vi "From Variant.vi"(0 "TTLController in":refnum<class "TTLController.lvclass">, 7 "Variant":variant, 9 "Prefix":string, 11 "error in (no error)":errorcluster) -> (4 "TTLController out":refnum<class "TTLController.lvclass">, 15 "error out":errorcluster)   [LabVIEW 2020, in "TTLController.lvclass"]
uses:
  TTLController.lvclass
  D:/Experiment VIs/Koop/KObject Class/KObject.lvclass
  epl-vi-lib/Koop/KObject Class/KObject.lvclass/KObject.ctl
  TTLController.lvclass/TTLController.ctl
  V0.ctl
  V2.ctl
  Trigger.ctl
  epl-vi-lib/Koop/KObject Class/Read Version.vi
  epl-vi-lib/Koop/KObject Class/KObject.lvclass
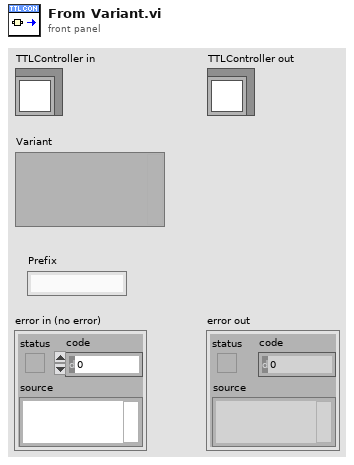
[diagram p1: front panel]
types:
  T1 = typedef "TTLController.lvclass/Serialized.ctl" = cluster{"Name":string, "Start":T2, "Stop":T2, "Pulse":cluster{"Active":bool, "IPI":string, "Width (ms)":dbl}}
  T2 = typedef "TTLController.lvclass/Trigger.ctl" = cluster{"When":string, "Expr":string}
  T3 = typedef "TTLController.lvclass/V0.ctl" = cluster{"Name":string, "Start":cluster{"When":string, "Value":dbl}, "Stop":cluster{"When":string, "Value":dbl}, "Pulse":cluster{"Active":bool, "Rate (Hz)":dbl, "Width (ms)":dbl}}
  T4 = typedef "TTLController.lvclass/V2.ctl" = cluster{"Name":string, "Start":T2, "Stop":T2, "Pulse":cluster{"Active":bool, "Rate (Hz)":dbl, "Width (ms)":dbl}}
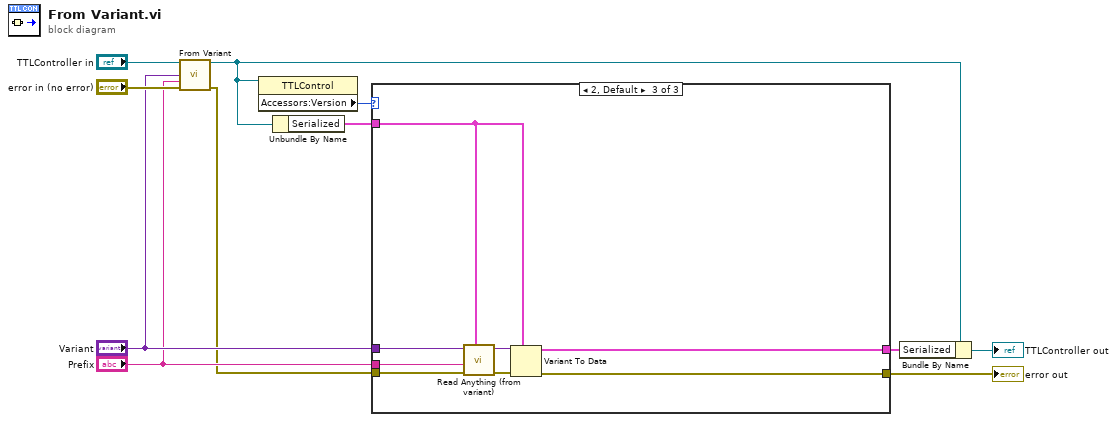
[diagram p0: block diagram]
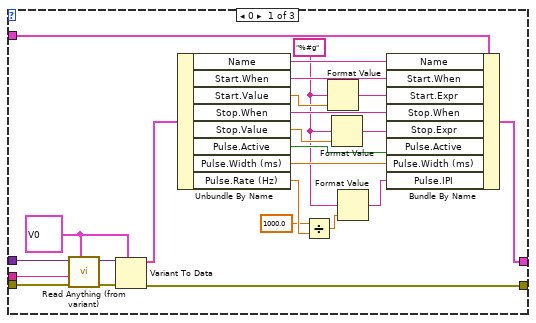
[diagram p2: hidden frame]
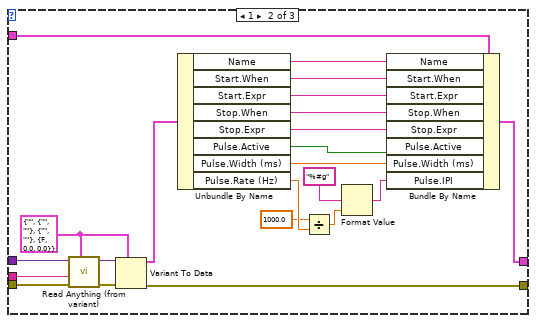
[diagram p3: hidden frame]
diagram:
  n1 = call-parent "From Variant.vi"("KObject in"="TTLController in", "Variant"="Variant", "Prefix"="Prefix", "error in (no error)"="error in (no error)") -> ("KObject out"=w2:refnum<class "TTLController.lvclass">, "error out"=w6:errorcluster)  [unwired: 10 in]
  n2 = property class="TTLControl"(reference=w2) -> ("Accessors:Version"=w3:i32)  [unwired: 1 in, 2 out]
  n3 = Unbundle By Name(w2) -> ("Serialized"=w1:T1)
  n4 = case shown="2, Default" w3 {
    tunnel: [w22 w46 w63] -> w9
    tunnel: "Variant" -> [w33 w55 w62]
    tunnel: "Prefix" -> [w32 w54 w61]
    tunnel: w6 -> [w31 w53 w60]
    tunnel: [w30 w52 w59] -> w5
    tunnel: w1 -> [w27 w49 w58]
    frame 0 {
      w12 = "%#g" ("string (\"\")")
      w29 = T3 {"Name"="", "Start"={"When"="Immediately", "Value"=0.0}, "Stop"={"When"="Delayed", "Value"=100.0}, "Pulse"={"Active"=FALSE, "Rate (Hz)"=0.0, "Width (ms)"=0.0}} ("V0")
      n5 = call "Read Anything (from variant).vi"("Type of Anything"=w29, "Error In"=w31, "Prefix"=w32, "Variant Database"=w33) -> ("Error Out"=w34:errorcluster, "Anything"=w35:variant)  [unwired: 5 in, 1 out]
      n6 = Variant To Data(error in=w34, type=w29, Variant=w35) -> (data=w28:T3, error out=w30:errorcluster)
      n7 = Unbundle By Name(w28) -> ("Name"=w26:string, "Start.When"=w25:string, "Start.Value"=w24:dbl, "Stop.When"=w21:string, "Stop.Value"=w20:dbl, "Pulse.Active"=w18:bool, "Pulse.Width (ms)"=w17:dbl, "Pulse.Rate (Hz)"=w16:dbl)
      n8 = Divide(x=1000.0, y=w16) -> (x/y=w14:dbl)
      n9 = Format Value(format string=w12, value (0)=w24) -> (output string=w23:string)  [unwired: 1 in]
      n10 = Format Value(format string=w12, value (0)=w20) -> (output string=w19:string)  [unwired: 1 in]
      n11 = Format Value(format string=w12, value (0)=w14) -> (output string=w13:string)  [unwired: 1 in]
      n12 = Bundle By Name(cluster=w27, "Name"=w26, "Start.When"=w25, "Start.Expr"=w23, "Stop.When"=w21, "Stop.Expr"=w19, "Pulse.Active"=w18, "Pulse.Width (ms)"=w17, "Pulse.IPI"=w13) -> (w22:T1)
    }
    frame 1 {
      w51 = T4 {"Name"="", "Start"={"When"="", "Expr"=""}, "Stop"={"When"="", "Expr"=""}, "Pulse"={"Active"=FALSE, "Rate (Hz)"=0.0, "Width (ms)"=0.0}} ("V0")
      n13 = call "Read Anything (from variant).vi"("Type of Anything"=w51, "Error In"=w53, "Prefix"=w54, "Variant Database"=w55) -> ("Error Out"=w56:errorcluster, "Anything"=w57:variant)  [unwired: 5 in, 1 out]
      n14 = Variant To Data(error in=w56, type=w51, Variant=w57) -> (data=w50:T4, error out=w52:errorcluster)
      n15 = Unbundle By Name(w50) -> ("Name"=w48:string, "Start.When"=w47:string, "Start.Expr"=w37:string, "Stop.When"=w45:string, "Stop.Expr"=w38:string, "Pulse.Active"=w44:bool, "Pulse.Width (ms)"=w43:dbl, "Pulse.Rate (Hz)"=w42:dbl)
      n16 = Divide(x=1000.0, y=w42) -> (x/y=w40:dbl)
      n17 = Format Value(format string="%#g" ("string (\"\")"), value (0)=w40) -> (output string=w39:string)  [unwired: 1 in]
      n18 = Bundle By Name(cluster=w49, "Name"=w48, "Start.When"=w47, "Start.Expr"=w37, "Stop.When"=w45, "Stop.Expr"=w38, "Pulse.Active"=w44, "Pulse.Width (ms)"=w43, "Pulse.IPI"=w39) -> (w46:T1)
    }
    frame 2, Default {
      n19 = call "Read Anything (from variant).vi"("Type of Anything"=w58, "Error In"=w60, "Prefix"=w61, "Variant Database"=w62) -> ("Error Out"=w64:errorcluster, "Anything"=w65:variant)  [unwired: 5 in, 1 out]
      n20 = Variant To Data(error in=w64, type=w58, Variant=w65) -> (data=w63:T1, error out=w59:errorcluster)
    }
  }
  "error out" <- w5
  n21 = Bundle By Name(cluster=w2, "Serialized"=w9) -> (→"TTLController out":refnum<class "TTLController.lvclass">)
